vi "CI_Dlg_More.vi"(8 "error in":errorcluster, 11 "Display State In":T1={"StandardColor"=0, "WarningColor"=15671808, "CriticalColor"=15671808, "Standard<>Warning Range"=0, "Warning<>Critical Range"=0}) -> (0 "error out":errorcluster, 2 "Cancel?":bool, 3 "Display State Out":T1={"StandardColor"=0, "WarningColor"=15671808, "CriticalColor"=15671808, "Standard<>Warning Range"=0, "Warning<>Critical Range"=0})   [LabVIEW 2010, in "CapacityIndicator.xctl"]
doc: "Copyright 2007 SAPHIR (Olivier JOURDAN) All Rights Reserved\n\nThis VI is the dialog box for the capacity indicator specifics properties in edition mode. It allows user to modify colors and threshold."
uses:
  CapacityIndicator.xctl
  CI_State.ctl
panel:
  in  "Cancel":bool
  in  "Ok":bool
  in  "Tab Control":enum32{"Thresholds and colors"}(tab)
  in  "Critical":u32(colorbox)
  in  "Warning":u32(colorbox)
  in  "Standard":u32(colorbox)
  in  "W<>C":u8=1 caption="Warning | Critical" min=1 max=100 step=1
  in  "S<>W":u8 caption="Standard | Warning" max=99 step=1
  # "Input"
  # "Output"
  # "Local"
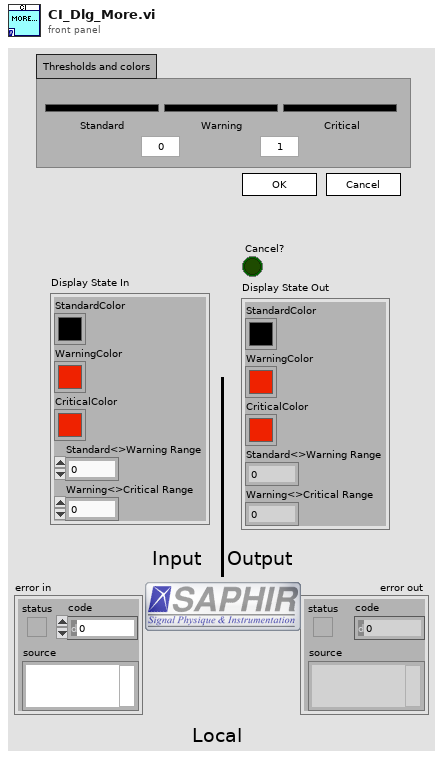
[diagram p1: front panel]
types:
  T1 = typedef "CapacityIndicator.xctl/CI_State.ctl" = cluster{"StandardColor":u32, "WarningColor":u32, "CriticalColor":u32, "Standard<>Warning Range":u8, "Warning<>Critical Range":u8}
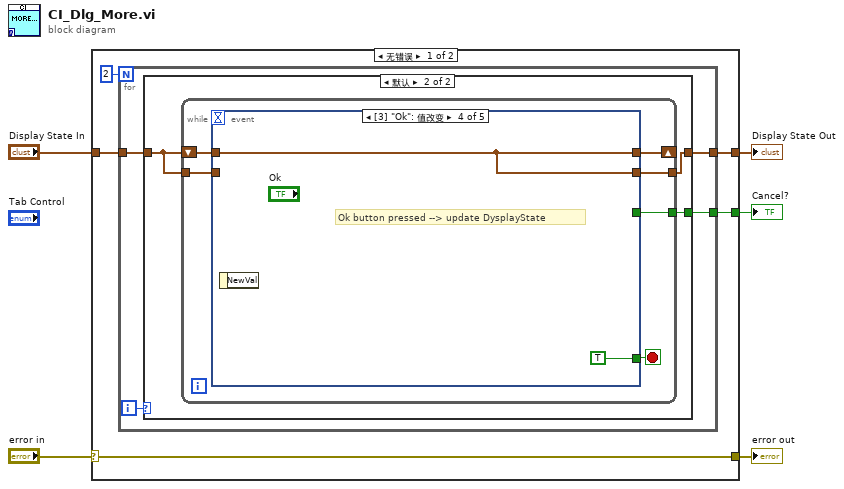
[diagram p0: block diagram]
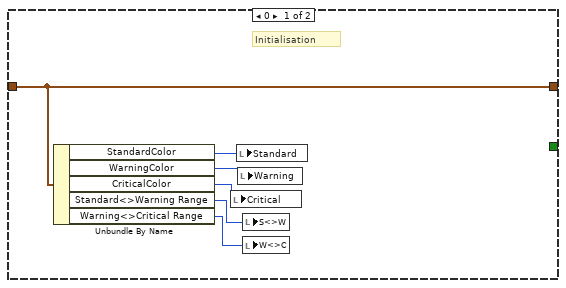
[diagram p2: hidden frame]
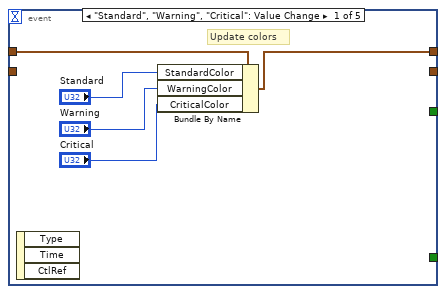
[diagram p3: hidden frame]
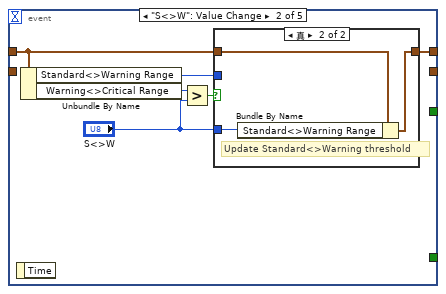
[diagram p4: hidden frame]
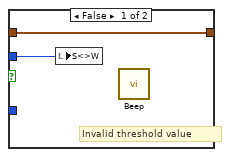
[diagram p5: hidden frame]
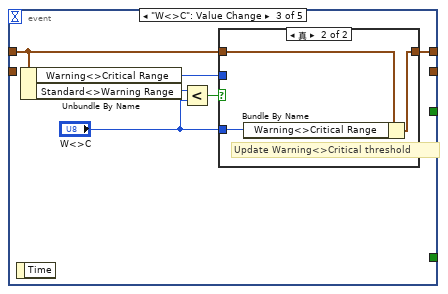
[diagram p6: hidden frame]
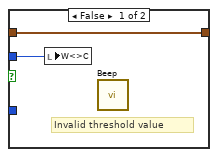
[diagram p7: hidden frame]
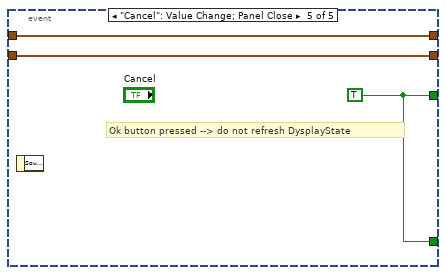
[diagram p8: hidden frame]
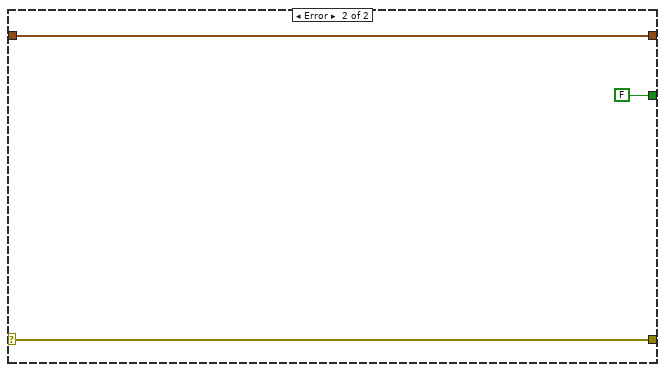
[diagram p9: hidden frame]
diagram:
  n1 = case shown="无错误" "error in" {
    selector: "error in" -> [w8 w64]
    tunnel: [w8 w64] -> w4
    tunnel: "Display State In" -> [w10 w63]
    tunnel: [w9 w63] -> w2
    tunnel: [w6 FALSE ("Cancel")] -> w1
    frame No Error {
      n2 = for {
        N: 2 -> [_]
        tunnel: w10 -> [w13]
        tunnel: [w12] -> w9
        tunnel: [w11] -> w6
        i -> [w14]
        n3 = case shown="默认" w14 {
          tunnel: w13 -> [w15 w23]
          tunnel: [w15 w22] -> w12
          tunnel: [_ w21] -> w11
          frame 0 {
            # "Initialisation"
            n4 = Unbundle By Name(w15) -> ("StandardColor"=w20:u32, "WarningColor"=w19:u32, "CriticalColor"=w18:u32, "Standard<>Warning Range"=w17:u8, "Warning<>Critical Range"=w16:u8)
            n5 = local write "Critical"(w18) -> ()
            n6 = local write "Standard"(w20) -> ()
            n7 = local write "Warning"(w19) -> ()
            n8 = local write "S<>W"(w17) -> ()
            n9 = local write "W<>C"(w16) -> ()
          }
          frame Default {
            n10 = while {
              shift-right: [w27] -> _
              shift-left: w23 -> [w29]
              tunnel: w23 -> [w25]
              tunnel: [w26] -> w22
              tunnel: [w24] -> w21
              stop <- w28 stop-if-true
              n11 = event shown="[3] \"Ok\": 值改变" {
                selector: _ -> [_ _ _ _ _]
                dyn-events: _ -> [_ _ _ _ _]
                timeout: _ -> [_ _ _ _ _]
                tunnel: w29 -> [w34 w40 w51 w57 w61]
                tunnel: [_ _ _ TRUE w59] -> w28
                tunnel: [w33 w39 w50 w57 w61] -> w27
                tunnel: [_ _ _ w57 w60] -> w26
                tunnel: w25 -> [_ _ _ _ w60]
                tunnel: [_ _ _ _ w59] -> w24
                event "Standard", "Warning", "Critical": Value Change {
                  # "Update colors"
                  n12 = event-data() -> ()  [unwired: 1 in, 3 out]
                  n13 = Bundle By Name(cluster=w34, "StandardColor"="Standard", "WarningColor"="Warning", "CriticalColor"="Critical") -> (w33:T1)
                }
                event "S<>W": Value Change {
                  n14 = event-data() -> ()  [unwired: 1 in, 1 out]
                  n15 = Unbundle By Name(w40) -> ("Standard<>Warning Range"=w35:u8, "Warning<>Critical Range"=w38:u8)
                  n16 = Greater?(x=w38, y="S<>W") -> (0:w37:bool)
                  n17 = case shown="真" w37 {
                    tunnel: w40 -> [w42 w45]
                    tunnel: [w42 w44] -> w39
                    tunnel: "S<>W" -> [_ w43]
                    tunnel: w35 -> [w41 _]
                    frame False {
                      # "Invalid threshold value"
                      n18 = local write "S<>W"(w41) -> ()
                      n19 = call <vilib>:"Beep.vi"() -> ()  [unwired: 12 in]
                    }
                    frame True {
                      # "Update Standard<>Warning threshold"
                      n20 = Bundle By Name(cluster=w45, "Standard<>Warning Range"=w43) -> (w44:T1)
                    }
                  }
                }
                event "W<>C": Value Change {
                  n21 = event-data() -> ()  [unwired: 1 in, 1 out]
                  n22 = Unbundle By Name(w51) -> ("Warning<>Critical Range"=w46:u8, "Standard<>Warning Range"=w49:u8)
                  n23 = Less?(x=w49, y="W<>C") -> (x < y?=w48:bool)
                  n24 = case shown="真" w48 {
                    tunnel: w51 -> [w53 w56]
                    tunnel: [w53 w54] -> w50
                    tunnel: "W<>C" -> [_ w55]
                    tunnel: w46 -> [w52 _]
                    frame False {
                      # "Invalid threshold value"
                      n25 = local write "W<>C"(w52) -> ()
                      n26 = call <vilib>:"Beep.vi"() -> ()  [unwired: 12 in]
                    }
                    frame True {
                      # "Update Warning<>Critical threshold"
                      n27 = Bundle By Name(cluster=w56, "Warning<>Critical Range"=w55) -> (w54:T1)
                    }
                  }
                }
                event "Ok": Value Change {
                  # "Ok button pressed --> update DysplayState"
                  n28 = event-data() -> ()  [unwired: 1 in, 1 out]
                }
                event "Cancel": Value Change; Panel Close {
                  w59 = TRUE ("Cancel")
                  # "Ok button pressed --> do not refresh DysplayState"
                  n29 = event-data() -> ()  [unwired: 1 in, 1 out]
                }
              }
            }
          }
        }
      }
    }
    frame Error {
    }
  }
  "error out" <- w4
  "Display State Out" <- w2
  "Cancel?" <- w1
